vi "update_standard_values.vi"(8 "error in (no error)":errorcluster, 11 "PrepLineObject in":refnum<class "PrepLineObject.lvclass">) -> (0 "error out":errorcluster, 3 "PrepLineObject out":refnum<class "PrepLineObject.lvclass">)   [LabVIEW 2017]
doc: "checks whether or not the switch is a switch of a pipette (inner-switch).\nIf so using the dilution factor of the pipette the VI calculates the new isotope amounts in the standard hat is attached to that pipette"
uses:
  Classes/PrepLineObject/PrepLineObject.lvclass
  <vilib>/Utility/config.llb/Write Key (Double).vi
  Classes/Pipette/Pipette.lvclass
  Classes/Standard/Standard.lvclass
  <vilib>/Utility/config.llb/NI_LVConfig.lvlib
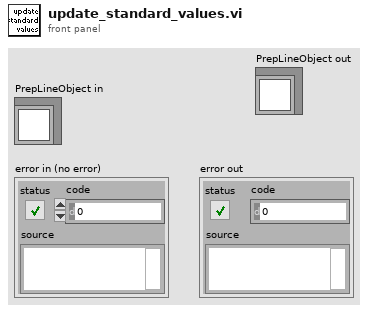
[diagram p1: front panel]
types:
  T1 = enum16{"fractional", "engineering", "exponential"}
  T2 = typedef "NI_LVConfig.lvlib/Config Data RefNum.ctl" = refnum<k1>
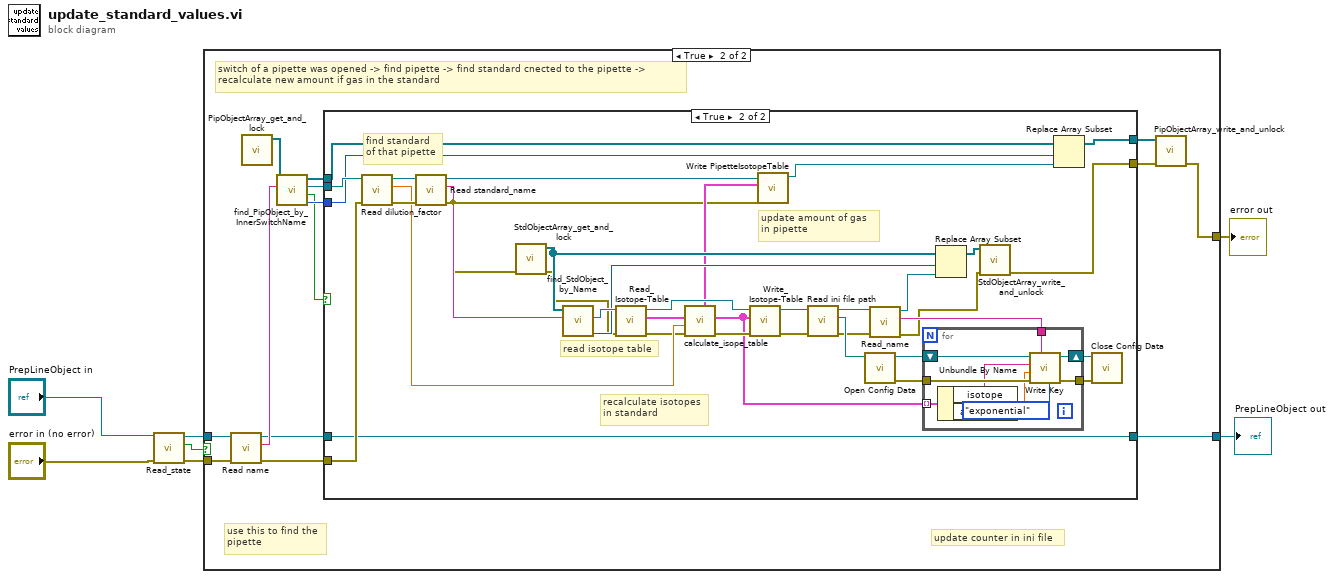
[diagram p0: block diagram]
diagram:
  n1 = call-dynamic "Read_state.vi"("error in (no error)"="error in (no error)", "PrepLineObject in"="PrepLineObject in") -> ("error out"=w6:errorcluster, "state"=w4:bool, "PrepLineObject out"=w5:refnum<class "PrepLineObject.lvclass">)  [unwired: 7 in]
  n2 = case shown="True" w4 {
    tunnel: [w9 w17] -> w7
    tunnel: w6 -> [w9 w21]
    tunnel: w5 -> [w8 w22]
    tunnel: [w8 w11] -> w1
    frame False {
      # "don't update"
    }
    frame True {
      # "use this to find the\npipette"
      # "update counter in ini file"
      # "switch of a pipette was opened -> find pipette -> find standard cnected to the pipette ->\nrecalculate new amount if gas in the standard"
      n3 = call-dynamic "Read name.vi"("error in (no error)"=w21, "PrepLineObject in"=w22) -> ("error out"=w18:errorcluster, "name"=w20:string, "PrepLineObject out"=w12:refnum<class "PrepLineObject.lvclass">)  [unwired: 7 in]
      n4 = call "PipObjectArray_get_and_lock.vi"() -> ("PipObjects"=w23:refnum<class "Pipette.lvclass">[])  [unwired: 10 in, 1 out]
      n5 = call "find_PipObject_by_InnerSwitchName.vi"("inner switch name"=w20, "PipObj Array in"=w23) -> ("index of Object in Array"=w14:i32, "found?"=w10:bool, "found PipObj out"=w19:refnum<class "Pipette.lvclass">, "PipObj Array out"=w15:refnum<class "Pipette.lvclass">[])  [unwired: 6 in]
      n6 = case shown="True" w10 {
        tunnel: w19 -> [_ w63]
        tunnel: w18 -> [w25 w56]
        tunnel: [w26 w34] -> w16
        tunnel: w15 -> [w26 w33]
        tunnel: w14 -> [_ w31]
        tunnel: [w25 w29] -> w13
        tunnel: w12 -> [w24 w27]
        tunnel: [w24 w27] -> w11
        frame False {
          # "this switch is not a pipette"
        }
        frame True {
          # "update amount of gas\nin pipette"
          # "recalculate isotopes\nin standard"
          # "read isotope table"
          # "find standard\nof that pipette"
          n7 = call-dynamic "Read dilution_factor.vi"("error in (no error)"=w56, "Pipette in"=w63) -> ("error out"=w57:errorcluster, "dilution_factor"=w51:dbl, "Pipette out"=w58:refnum<class "Pipette.lvclass">)  [unwired: 7 in]
          n8 = call-dynamic "Read standard_name.vi"("error in (no error)"=w57, "Pipette in"=w58) -> ("error out"=w28:errorcluster, "standard_name"=w54:string, "Pipette out"=w35:refnum<class "Pipette.lvclass">)  [unwired: 7 in]
          n9 = call "StdObjectArray_get_and_lock.vi"("error in (no error)"=w28) -> ("error out"=w36:errorcluster, "StandardObjects"=w44:refnum<class "Standard.lvclass">[])  [unwired: 9 in]
          n10 = call "find_StdObject_by_Name.vi"("std_name"=w54, "StdObj Array in"=w44) -> ("index of Object in Array"=w45:i32, "found StdObj out"=w55:refnum<class "Standard.lvclass">)  [unwired: 6 in, 2 out]
          n11 = call-dynamic "Read_Isotope-Table.vi"("error in (no error)"=w36, "Standard in"=w55) -> ("error out"=w50:errorcluster, "Isotope Table"=w52:cluster{"isotope":string, "amount cc":dbl}[], "Standard out"=w49:refnum<class "Standard.lvclass">)  [unwired: 7 in]
          n12 = call "calculate_isope_table.vi"("error in (no error)"=w50, "dilution_factor"=w51, "Isotope Table"=w52) -> ("error out"=w48:errorcluster, "Isotope Table new"=w39:cluster{"isotope":string, "amount cc":dbl}[], "PipetteIsotopeTable"=w30:cluster{"isotope":string, "amount cc":dbl}[])  [unwired: 6 in]
          n13 = call-dynamic "Write_Isotope-Table.vi"("error in (no error)"=w48, "Isotope Table"=w39, "Standard in"=w49) -> ("error out"=w46:errorcluster, "Standard out"=w47:refnum<class "Standard.lvclass">)  [unwired: 7 in]
          n14 = call-dynamic "Write PipetteIsotopeTable.vi"("error in (no error)"=w28, "PipetteIsotopeTable"=w30, "Pipette in"=w35) -> ("Pipette out"=w32:refnum<class "Pipette.lvclass">)  [unwired: 7 in, 1 out]
          n15 = call-dynamic "Read ini file path.vi"("error in (no error)"=w46, "Standard in"=w47) -> ("error out"=w41:errorcluster, "ini file path"=w43:path, "Standard out"=w42:refnum<class "Standard.lvclass">)  [unwired: 7 in]
          n16 = call <vilib>:"Open Config Data.vi"("configuration file path"=w43) -> ("error out"=w62:errorcluster, "refnum"=w61:T2)  [unwired: 8 in, 1 out]
          n17 = call-dynamic "Read_name.vi"("error in (no error)"=w41, "Standard in"=w42) -> ("error out"=w38:errorcluster, "standard name"=w40:string, "Standard out"=w37:refnum<class "Standard.lvclass">)  [unwired: 7 in]
          n18 = for {
            tunnel: w62 -> [w72]
            tunnel: [w70] -> w60
            tunnel: w40 -> [w68]
            tunnel: w39 -> [w67] mode=indexing
            shift-right: [w69] -> w59
            shift-left: w61 -> [w71]
            n19 = Unbundle By Name(w67) -> ("isotope"=w66:string, "amount cc"=w65:dbl)
            n20 = call-poly <vilib>:"Write Key.vi"("format (fractional)"=T1."exponential", "section"=w68, "error in (no error)"=w72, "value"=w65, "key"=w66, "refnum"=w71) -> ("error out"=w70:errorcluster, "refnum out"=w69:T2)  [unwired: 3 in, 1 out]
          }
          n21 = Replace Array Subset(array=w44, new element=w37, index=w45) -> (w53:refnum<class "Standard.lvclass">[])
          n22 = call "StdObjectArray_write_and_unlock.vi"("error in (no error)"=w38, "StandardObjects"=w53) -> ("error out"=w29:errorcluster)  [unwired: 9 in]
          n23 = Replace Array Subset(array=w33, new element=w32, index=w31) -> (w34:refnum<class "Pipette.lvclass">[])
          n24 = call <vilib>:"Close Config Data.vi"("error in (no error)"=w60, "refnum"=w59) -> ()  [unwired: 8 in, 2 out]
        }
      }
      n25 = call "PipObjectArray_write_and_unlock.vi"("error in (no error)"=w13, "PipObjects"=w16) -> ("error out"=w17:errorcluster)  [unwired: 9 in]
    }
  }
  "error out" <- w7
  "PrepLineObject out" <- w1
